vi "check 5 phase.vi"(0 "LstBox Refnum":refnum<vi>, 1 "AD F/P Array":dbl[][](array[numeric]), 2 "10R F/P Array":dbl[][](array[numeric]), 3 "1R F/P Array":dbl[][](array[numeric]), 4 "Wagner F/P Array":dbl[][](array[numeric]), 5 "Kelvin F/P Array":dbl[][](array[numeric]), 6 "Direnc 1 - Direnc 2":u16(ring)=2 items=["1M(Ohm) / 100K(Ohm)", "100K(Ohm) / 10K(Ohm)", "10K(Ohm) / 1K(Ohm)", "1K(Ohm) / 100(Ohm)", "100(Ohm) / 10(Ohm)", "10(Ohm) / 1(Ohm)"], 7 "Frekanslar":dbl[](array[numeric]), 9 "frekans index":dbl) -> (14 "logical AND":bool)   [LabVIEW 2014]
panel:
  out "Array":bool[](array[boolean])
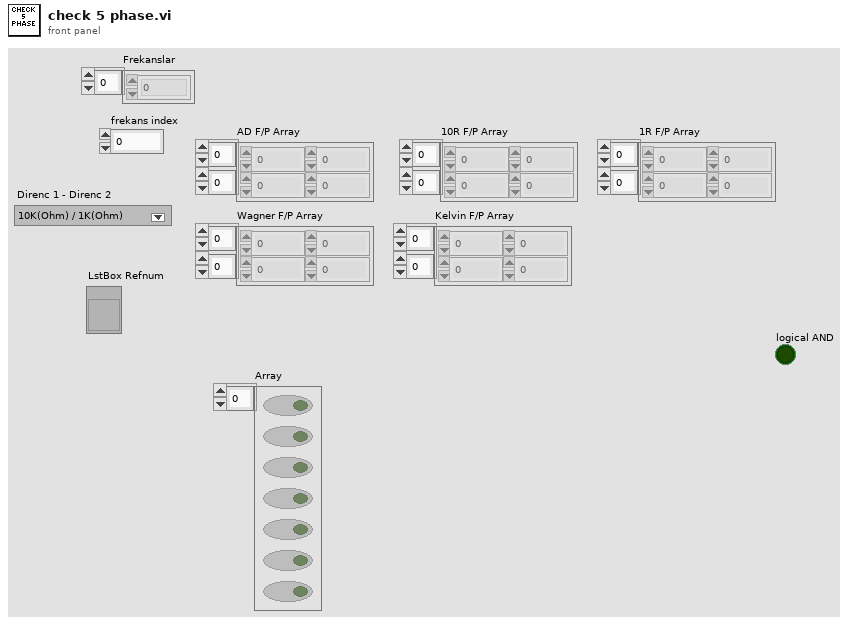
[diagram p1: front panel]
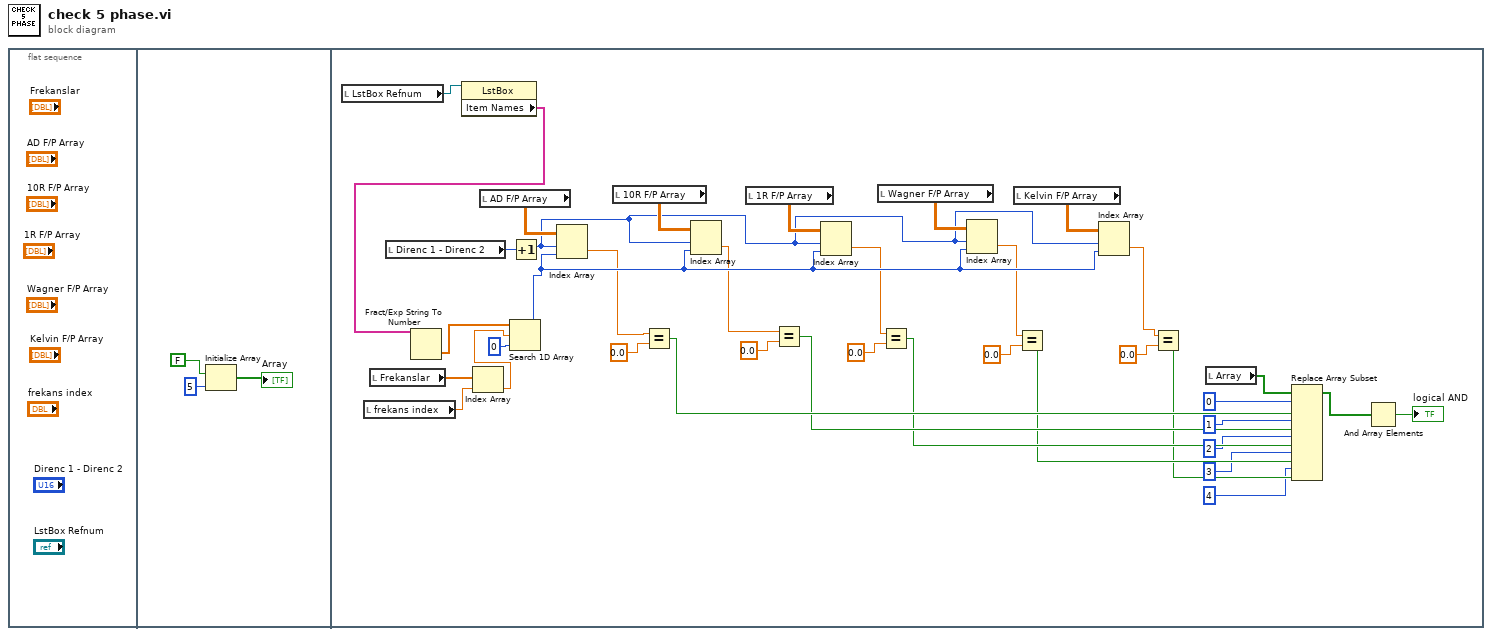
[diagram p0: block diagram]
diagram:
  n1 = flat-sequence {
    frame #0 {
    }
    frame #1 {
      n2 = Initialize Array(FALSE, 5 ("dimension size")) -> (→"Array":bool[])
    }
    frame #2 {
      n3 = local read "LstBox Refnum"() -> (w34:refnum<vi>)
      n4 = local read "frekans index"() -> (w38:dbl)
      n5 = local read "Frekanslar"() -> (w37:dbl[])
      n6 = local read "Direnc 1 - Direnc 2"() -> (w36:u16)
      n7 = property class="LstBox"(reference=w34) -> ("Item Names"=w33:string[])  [unwired: 1 in, 2 out]
      n8 = Fract/Exp String To Number(string=w33) -> (number=w39:dbl[])  [unwired: 3 in, 1 out]
      n9 = Index Array(array=w37, index=w38) -> (element=w41:dbl)
      n10 = local read "AD F/P Array"() -> (w35:dbl[][])
      n11 = Search 1D Array(1D array=w39, element=w41, start index (0)=0) -> (index of element=w27:i32)
      n12 = Increment(x=w36) -> (x+1=w28:u16)
      n13 = Index Array(array=w35, index (row)=w28, index (col)=w27) -> (element=w26:dbl)
      n14 = local read "10R F/P Array"() -> (w32:dbl[][])
      n15 = Equal?(x=w26, y=0.0) -> (x = y?=w14:bool)
      n16 = Index Array(array=w32, index (row)=w28, index (col)=w27) -> (element=w20:dbl)
      n17 = local read "1R F/P Array"() -> (w31:dbl[][])
      n18 = Equal?(x=w20, y=0.0) -> (x = y?=w13:bool)
      n19 = Index Array(array=w31, index (row)=w28, index (col)=w27) -> (element=w19:dbl)
      n20 = local read "Wagner F/P Array"() -> (w30:dbl[][])
      n21 = Equal?(x=w19, y=0.0) -> (x = y?=w12:bool)
      n22 = Index Array(array=w30, index (row)=w28, index (col)=w27) -> (element=w18:dbl)
      n23 = local read "Kelvin F/P Array"() -> (w29:dbl[][])
      n24 = Equal?(x=w18, y=0.0) -> (x = y?=w11:bool)
      n25 = Index Array(array=w29, index (row)=w28, index (col)=w27) -> (element=w17:dbl)
      n26 = Equal?(x=w17, y=0.0) -> (x = y?=w10:bool)
      n27 = local read "Array"() -> (w16:bool[])
      n28 = Replace Array Subset(array=w16, new element #1=w14, index #1=0, new element #2=w13, index #2=1, new element #3=w12, index #3=2, new element #4=w11, index #4=3, new element #5=w10, index #5=4) -> (w15:bool[])
      n29 = And Array Elements(Boolean array=w15) -> (logical AND=→"logical AND":bool)
    }
  }
